vi "Labview to GMAIL.vi"() -> ()   [LabVIEW 2021]
uses:
  <vilib>/smtpClient/Set Message Text.vi
  <vilib>/smtpClient/LabVIEWSMTPClient.lvlib
panel:
  in  "attachments":path[](array[path])
  in  "password":string
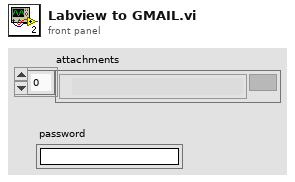
[diagram p1: front panel]
types:
  T1 = typedef "LabVIEWSMTPClient.lvlib/SmtpClientHandle.ctl" = refnum<k1>
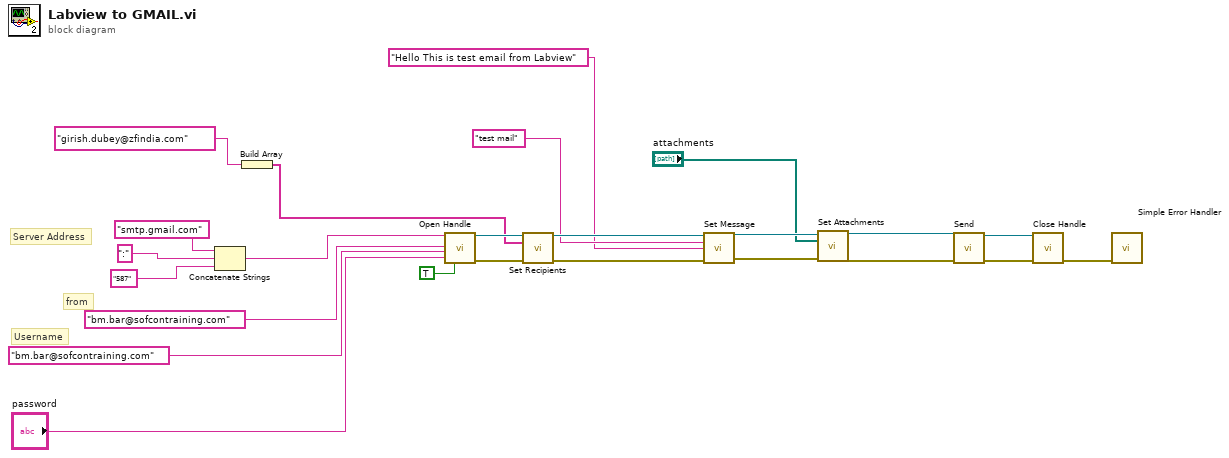
[diagram p0: block diagram]
diagram:
  # "Server Address"
  # "from"
  # "Username"
  n1 = Concatenate Strings "Concatenate Strings"("smtp.gmail.com" ("string"), ":" ("string"), "587" ("string")) -> (w14:string)
  n2 = Build Array "Build Array"("girish.dubey@zfindia.com" ("from")) -> (w9:string[])
  n3 = call <vilib>:"Open Handle.vi"("server address"=w14, "from"="bm.bar@sofcontraining.com", "username"="bm.bar@sofcontraining.com", "password"="password", "use TLS (false)"=TRUE) -> ("handle out"=w24:T1, "error out"=w18:errorcluster)  [unwired: 9 in]
  n4 = call <vilib>:"Set Recipients.vi"("handle in"=w24, "to"=w9, "error in (no error)"=w18) -> ("handle out"=w23:T1, "error out"=w19:errorcluster)  [unwired: 11 in]
  n5 = call-poly <vilib>:"Set Message.vi"("handle in"=w23, "subject"="test mail", "plain text message"="Hello This is test email from Labview", "error in (no error)"=w19) -> ("handle out"=w7:T1, "error out"=w4:errorcluster)  [unwired: 10 in]
  n6 = call <vilib>:"Set Attachments.vi"("handle in"=w7, "attachments"="attachments", "error in (no error)"=w4) -> ("handle out"=w6:T1, "error out"=w5:errorcluster)  [unwired: 11 in]
  n7 = call <vilib>:"Send.vi"("handle in"=w6, "error in (no error)"=w5) -> ("handle out"=w22:T1, "error out"=w20:errorcluster)  [unwired: 11 in, 1 out]
  n8 = call <vilib>:"Close Handle.vi"("handle in"=w22, "error in (no error)"=w20) -> ("error out"=w21:errorcluster)  [unwired: 12 in, 1 out]
  n9 = call <vilib>:"Simple Error Handler.vi"("error in (no error)"=w21) -> ()  [unwired: 4 in, 5 out]
